vi "Graph_Any_ERD_ Read_ List.vi"(0 "GEA2 Reference In":refnum<k24>, 5 "GEA Inputs":T2={"Source"=229, "Destination"=36} {"Destination" format="%.0x"; "Source" format="%.0x"}, 9 "ERD Graph Cntrl":T3={"ERD 3"={"ERD #"=0, "Data Type"=enum."uint16_t", "Scaler"=1}, "ERD 2"={"ERD #"=0, "Data Type"=enum."uint16_t", "Scaler"=1}, "ERD 1"={"ERD #"=0, "Data Type"=enum."uint16_t", "Scaler"=1}} {"ERD 1"."Scaler" min=1; "ERD 1"."ERD #" format="%.0x"; "ERD 2"."Scaler" min=1; "ERD 2"."ERD #" format="%.0x"; "ERD 3"."Scaler" min=1; "ERD 3"."ERD #" format="%.0x"}, 11 "Error In":errorcluster) -> (4 "GEA2 Reference Out":refnum<k24>, 6 "ERD Graph  Ind":T1, 15 "Error Out":errorcluster)   [LabVIEW 2023]
uses:
  type defs/ERD_Graph_All.ctl
  type defs/ERD_Graph.ctl
  Common/LabVIEW GEA2 Toolkit/GEA3/type defs/Data Type.ctl
  D:/Common/LabVIEW GEA2 Toolkit/source/GEA3 DLL Source/GeaCommunication.dll
  Common/LabVIEW GEA2 Toolkit/source/GEA3 DLL Source/GeaCommunication.dll
  Common/LabVIEW GEA2 Toolkit/GEA3/type defs/Source_Destination.ctl
  Common/LabVIEW GEA2 Toolkit/GEA3/type defs/ERD Read Data In.ctl
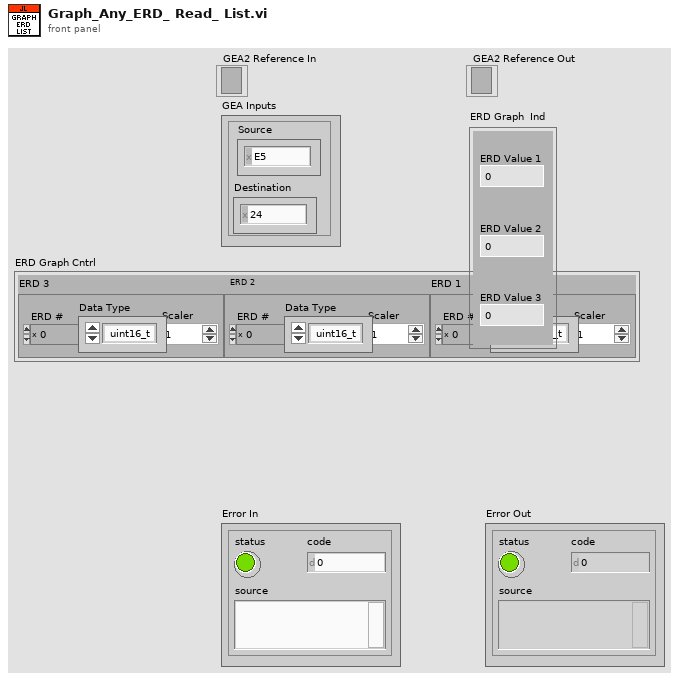
[diagram p1: front panel]
types:
  T1 = cluster{"ERD Value 1":dbl, "ERD Value 2":dbl, "ERD Value 3":dbl}
  T2 = typedef "Source_Destination.ctl" = cluster{"Source":u8, "Destination":u8}
  T3 = typedef "ERD_Graph_All.ctl" = cluster{"ERD 3":T4, "ERD 2":T4, "ERD 1":T4}
  T4 = typedef "ERD_Graph.ctl" = cluster{"ERD #":u16, "Data Type":T5, "Scaler":u32}
  T5 = typedef "Data Type.ctl" = enum16{"string", "boolean", "uint8_t", "uint16_t", "uint32_t", "uint64_t", "int8_t", "int16_t", "int32_t", "int64_t"}
  T6 = typedef "ERD Read Data In.ctl" = cluster{"ERD Number":u16, "Data Type":enum16{"string", "boolean", "uint8_t", "uint16_t", "uint32_t", "uint64_t", "int8_t", "int16_t", "int32_t", "int64_t"}}
  T7 = typedef "ERD Read Data Out.ctl" = cluster{"ERD Number":u16, "Data":string}
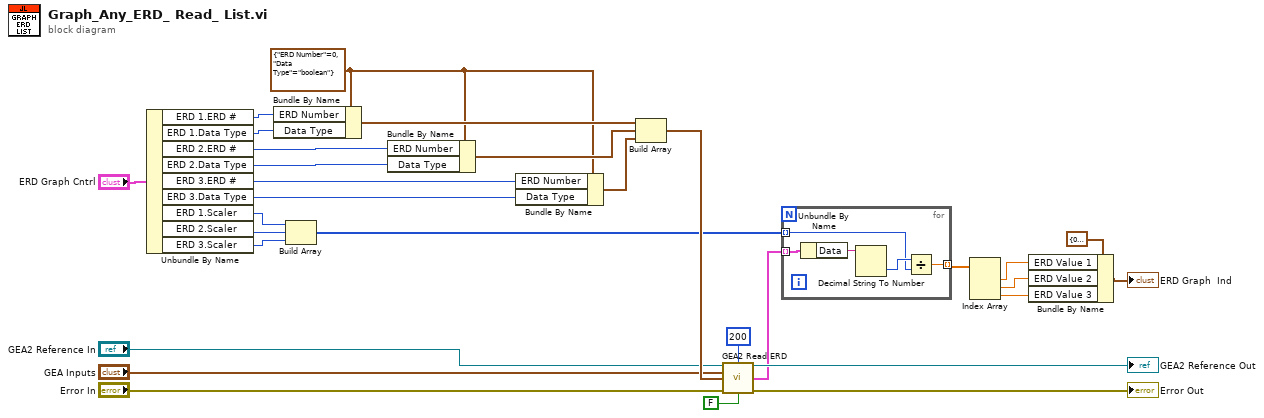
[diagram p0: block diagram]
diagram:
  w26 = T6 {"ERD Number"=0, "Data Type"=enum."boolean"} ("ERD Read Data In 2")
  n1 = Unbundle By Name("ERD Graph Cntrl") -> ("ERD 1.ERD #"=w20:u16, "ERD 1.Data Type"=w21:T5, "ERD 2.ERD #"=w22:u16, "ERD 2.Data Type"=w23:T5, "ERD 3.ERD #"=w24:u16, "ERD 3.Data Type"=w25:T5, "ERD 1.Scaler"=w13:u32, "ERD 2.Scaler"=w12:u32, "ERD 3.Scaler"=w11:u32)
  n2 = Bundle By Name(cluster=w26, "ERD Number"=w20, "Data Type"=w21) -> (w27:T6)
  n3 = Build Array(w13, w12, w11) -> (w10:u32[])
  n4 = Bundle By Name(cluster=w26, "ERD Number"=w22, "Data Type"=w23) -> (w28:T6)
  n5 = Bundle By Name(cluster=w26, "ERD Number"=w24, "Data Type"=w25) -> (w29:T6)
  n6 = Build Array(w27, w28, w29) -> (w19:T6[])
  n7 = call "GEA2 Read ERD.vi"("GEA2 Reference In"="GEA2 Reference In", "Read Timeout (ms)"=u32 200, "GEA Inputs"="GEA Inputs", "Read ERD List"=w19, "Error In"="Error In", "Verify ERD Response?"=FALSE) -> ("GEA2 Reference Out"=→"GEA2 Reference Out":refnum<k24>, "ERD Data Out"=w9:T7[], "Error Out"=→"Error Out":errorcluster)  [unwired: 6 in, 1 out]
  n8 = for {
    tunnel: w10 -> [w32] mode=indexing
    tunnel: w9 -> [w35] mode=indexing
    tunnel: [w31] -> w8 mode=indexing
    n9 = Unbundle By Name(w35) -> ("Data"=w34:string)
    n10 = Decimal String To Number(string=w34) -> (number=w33:i32)  [unwired: 2 in, 1 out]
    n11 = Divide(x=w33, y=w32) -> (x/y=w31:dbl)
  }
  n12 = Index Array(array=w8) -> (element #1=w6:dbl, element #2=w5:dbl, element #3=w4:dbl)  [unwired: 3 in]
  n13 = Bundle By Name(cluster=T1 {"ERD Value 1"=0.0, "ERD Value 2"=0.0, "ERD Value 3"=0.0} ("ERD Graph  Ind"), "ERD Value 1"=w6, "ERD Value 2"=w5, "ERD Value 3"=w4) -> (→"ERD Graph  Ind":T1)
